vi "总磷氨氮通讯.vi"() -> ()   [LabVIEW 2016, in "斯坦道仪器.lvlib"]
uses:
  <vilib>/Plasmionique/MB Master/MB_Master_Serial/MB_Master_Serial.lvclass
  D:/Program Files (x86)/National Instruments/LabVIEW 2016/vi.lib/Plasmionique/MB Master/MB_Master/MB_Master.lvclass
  <vilib>/Utility/config.llb/Write Key (Boolean).vi
  <vilib>/Utility/config.llb/Write Key (String).vi
  <vilib>/Utility/config.llb/Read Key (Boolean).vi
  <vilib>/Utility/config.llb/Read Key (String).vi
  <vilib>/Plasmionique/MB Master/MB_Master/MB_Master.lvclass
  <vilib>/Utility/config.llb/NI_LVConfig.lvlib
  <vilib>/Plasmionique/MB Master/MB Master.lvlib
  <vilib>/ptbypt/NI_PtbyPt.lvlib
panel:
  out "量程":u16
  out "序列号":string
  out "状态告警区":T1
  out "测量数据区":T2 {"单位" items=["ug/L", "mg/L", "ppm", "mg/m3", "cm", "ppb", "ug/m3", "%", "nmol/mol", "umol/mol", "MPN/L", "MPN/100ml", "ng/m3", "NTU", "无量纲", "ms/cm", "us/cm", "℃", "mV", "万个/L"]}
  out "status":bool
  out "关键参数区":T3
  in  "读关键参数区":bool
  in  "读状态告警区":bool
  in  "读测量数据区":bool
  in  "站号":u16(ring) items=["总磷"=1, "氨氮"=3]
  in  "停止":bool
  in  "启动":bool
  in  "控制命令":u16(ring) items=["启动测量"=1, "标样核查"=2, "零点核查"=3, "跨度核查"=4, "空白测试"=5, "平行样测试"=6, "加标回收"=7, "空白校准"=8, "标样校准"=9, "初始化（清洗）"=10, "停止测试"=11, "仪器重启"=12, "校时"=13, "模式设置"=14, "测量间隔设置"=15]
  in  "控制命令参数":u16[](array[numeric]) format="%04xH"
  in  "VISA Resource":refnum<visa-resource-name>
  in  "启用模块":bool
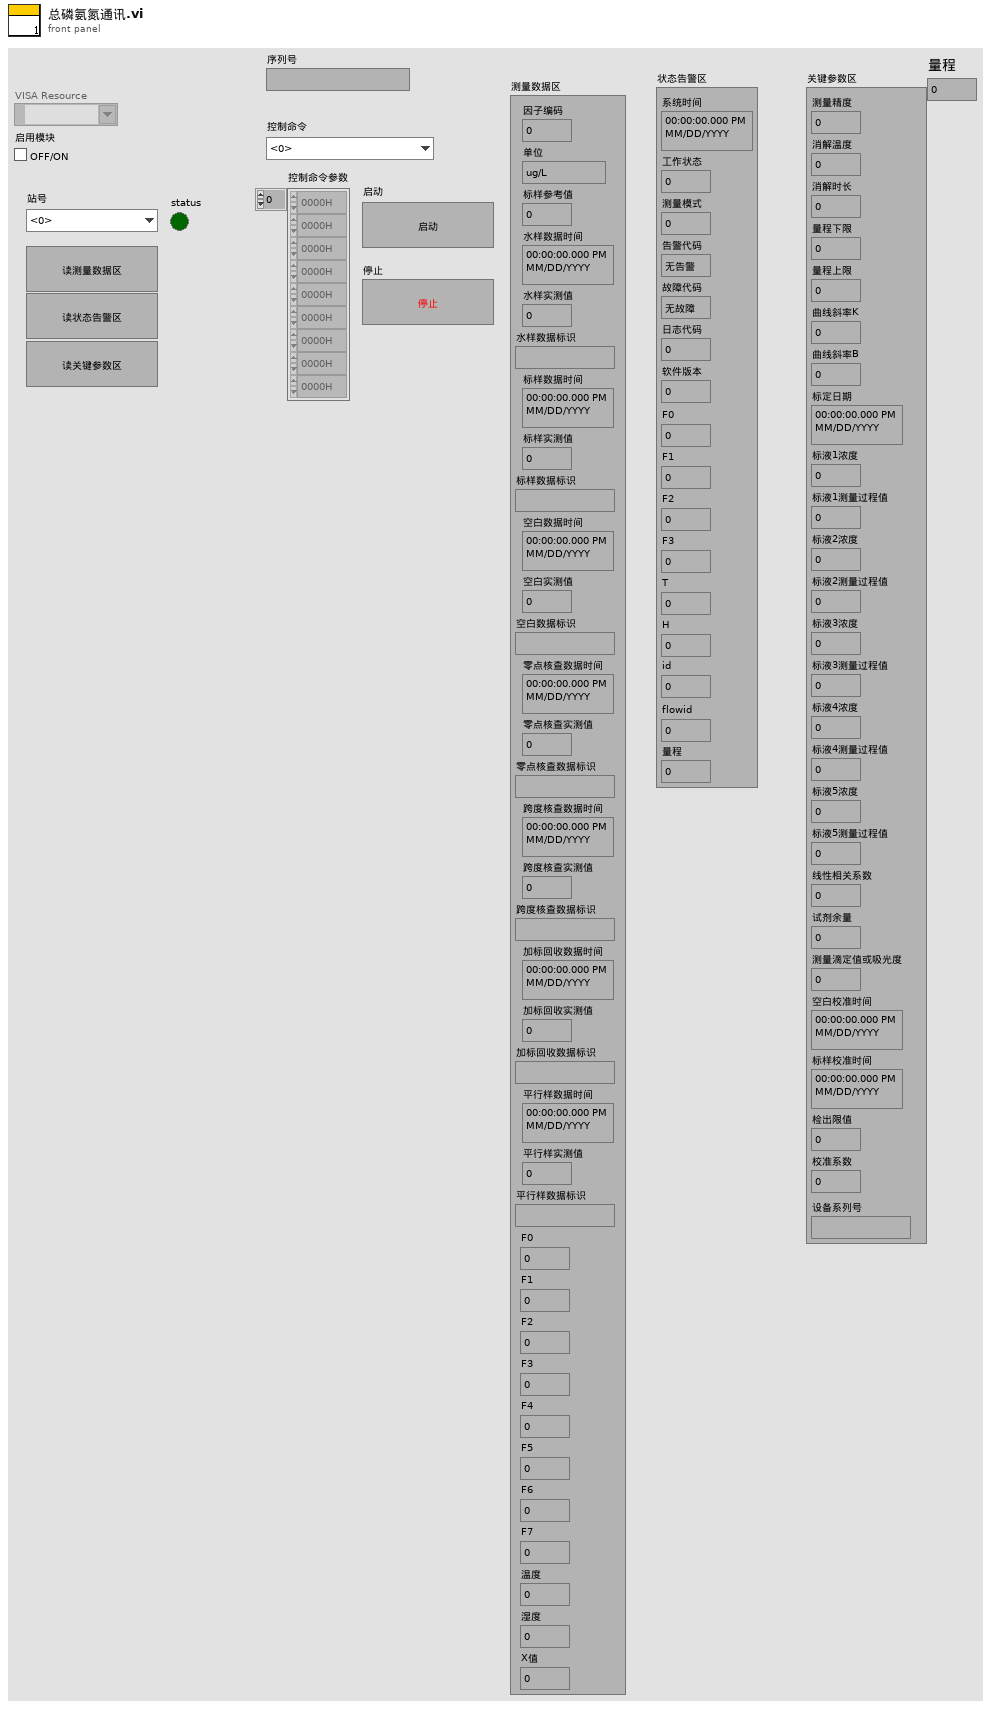
[diagram p1: front panel]
types:
  T1 = cluster{"系统时间":timestamp, "工作状态":u16, "测量模式":u16, "告警代码":enum16{"无告警", "缺试剂告警", "缺水样告警", "缺蒸馏水告警", "缺标液告警", "仪表漏液告警", "标定异常告警", "超量程告警", "加热异常", "低试剂预警", "超上限告警", "超下限告警", "仪表内部其他异常", "滴定异常告警", "电极异常告警", "量程切换告警", "参数设置告警", "PH电极电位异常", "电导率电极异常", "浊度光度异常", "溶解氧电极异常", "溶解氧光强异常", "温度异常告警", "PH异常告警", "溶解氧异常告警", "电导率异常告警", "浊度异常告警", "叶绿素异常告警", "藻密度异常告警", "蓝绿藻异常告警", "ORP异常告警", "氨氮异常告警", "清洁刷异常告警", "SD卡异常告警", "蓝牙异常告警", "Wifi异常告警", "流程异常告警"}, "故障代码":enum16{"无故障", "电机故障", "温度故障", "通讯故障", "滴定故障"}, "日志代码":u16, "软件版本":u16, "F0":sgl, "F1":sgl, "F2":sgl, "F3":sgl, "T":sgl, "H":sgl, "id":u16, "flowid":u16, "量程":u16}
  T2 = cluster{"因子编码":u32, "单位":u16, "标样参考值":sgl, "水样数据时间":timestamp, "水样实测值":sgl, "水样数据标识":string, "标样数据时间":timestamp, "标样实测值":sgl, "标样数据标识":string, "空白数据时间":timestamp, "空白实测值":sgl, "空白数据标识":string, "零点核查数据时间":timestamp, "零点核查实测值":sgl, "零点核查数据标识":string, "跨度核查数据时间":timestamp, "跨度核查实测值":sgl, "跨度核查数据标识":string, "加标回收数据时间":timestamp, "加标回收实测值":sgl, "加标回收数据标识":string, "平行样数据时间":timestamp, "平行样实测值":sgl, "平行样数据标识":string, "F0":sgl, "F1":sgl, "F2":sgl, "F3":sgl, "F4":sgl, "F5":sgl, "F6":sgl, "F7":sgl, "温度":sgl, "湿度":sgl, "X值":sgl}
  T3 = cluster{"测量精度":u16, "消解温度":u16, "消解时长":u16, "量程下限":sgl, "量程上限":sgl, "曲线斜率K":sgl, "曲线斜率B":sgl, "标定日期":timestamp, "标液1浓度":sgl, "标液1测量过程值":sgl, "标液2浓度":sgl, "标液2测量过程值":sgl, "标液3浓度":sgl, "标液3测量过程值":sgl, "标液4浓度":sgl, "标液4测量过程值":sgl, "标液5浓度":sgl, "标液5测量过程值":sgl, "线性相关系数":sgl, "试剂余量":u32, "测量滴定值或吸光度":sgl, "空白校准时间":timestamp, "标样校准时间":timestamp, "检出限值":sgl, "校准系数":sgl, "设备系列号":string}
  T4 = cluster{"系统时间":timestamp, "工作状态":enum16{"空闲", "水样测试", "标样核查", "零点核查", "跨度核查", "空白测试", "平行样测试", "加标回收", "空白校准", "标样校准", "初始化（清洗）"}, "测量模式":enum16{"待机", "连续模式", "周期模式", "定点模式", "受控模式", "手动模式"}, "告警代码":enum16{"无告警", "缺试剂告警", "缺水样告警", "缺蒸馏水告警", "缺标液告警", "仪表漏液告警", "标定异常告警", "超量程告警", "加热异常", "低试剂预警", "超上限告警", "超下限告警", "仪表内部其他异常", "滴定异常告警", "电极异常告警", "量程切换告警", "参数设置告警", "PH电极电位异常", "电导率电极异常", "浊度光度异常", "溶解氧电极异常", "溶解氧光强异常", "温度异常告警", "PH异常告警", "溶解氧异常告警", "电导率异常告警", "浊度异常告警", "叶绿素异常告警", "藻密度异常告警", "蓝绿藻异常告警", "ORP异常告警", "氨氮异常告警", "清洁刷异常告警", "SD卡异常告警", "蓝牙异常告警", "Wifi异常告警", "流程异常告警"}, "故障代码":enum16{"无故障", "电机故障", "温度故障", "通讯故障", "滴定故障"}, "日志代码":u16, "软件版本":u16, "F0":sgl, "F1":sgl, "F2":sgl, "F3":sgl, "T":sgl, "H":sgl, "id":u16, "flowid":u16, "量程":u16}
  T5 = typedef "NI_LVConfig.lvlib/Config Data RefNum.ctl" = refnum<k1>
  T6 = enum8{"Enabled", "Disabled", "Disabled and Grayed Out"}
  T7 = cluster{"baud rate (bps)":u32, "stop bits":u16, "parity":u16, "flow control":u16, "timeout":u32, "retries":i32}
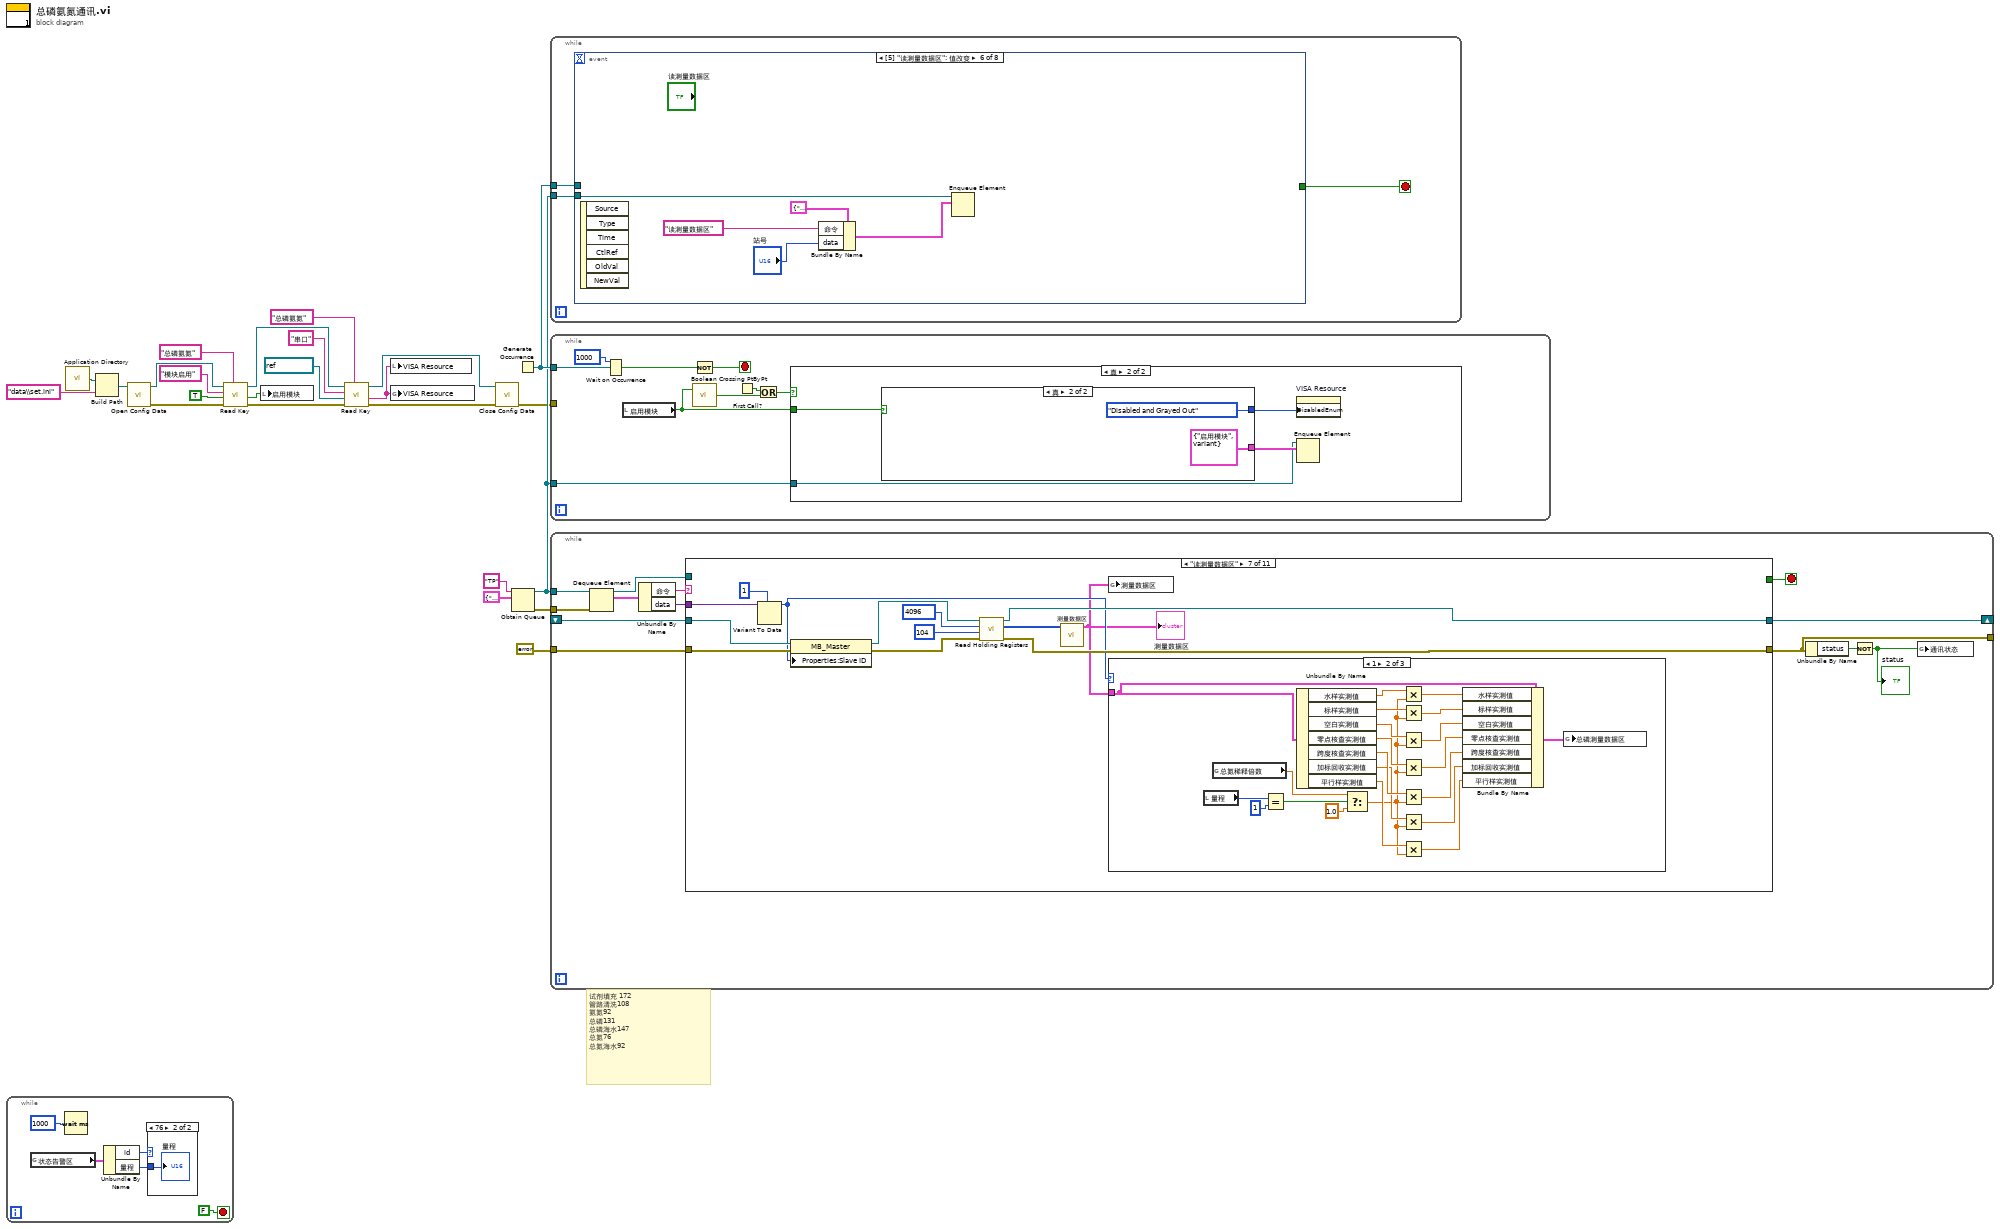
[diagram p0: block diagram]
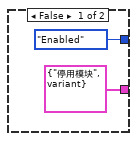
[diagram p4: hidden frame]
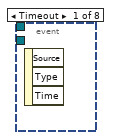
[diagram p5: hidden frame]
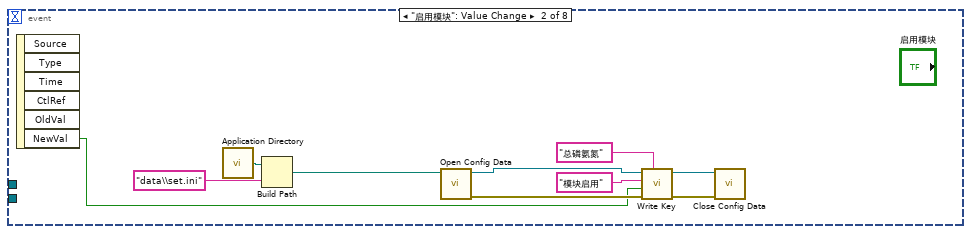
[diagram p6: hidden frame]
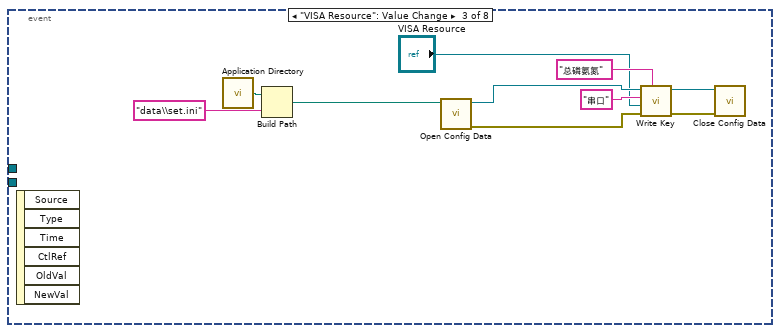
[diagram p7: hidden frame]
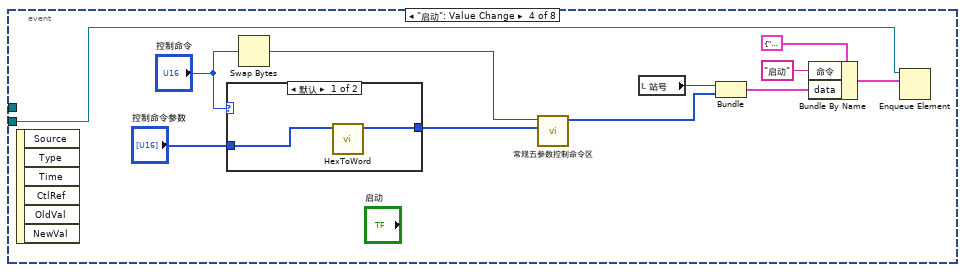
[diagram p8: hidden frame]
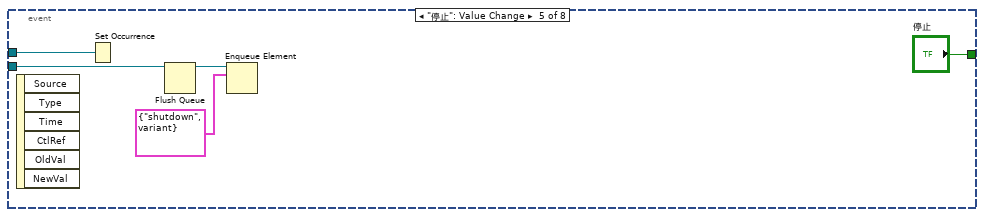
[diagram p10: hidden frame]
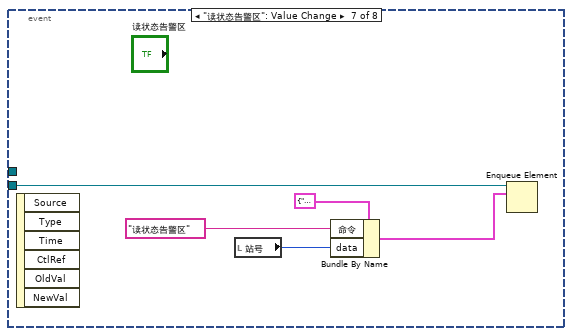
[diagram p11: hidden frame]
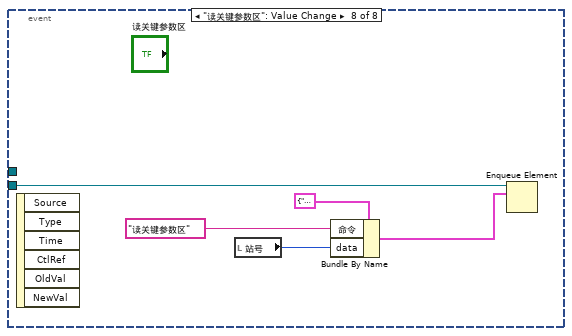
[diagram p12: hidden frame]
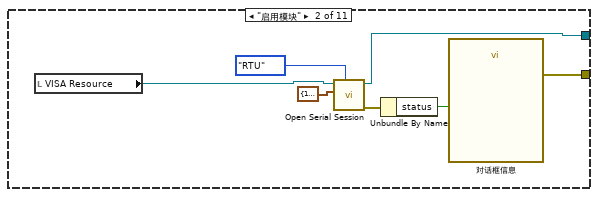
[diagram p14: hidden frame]
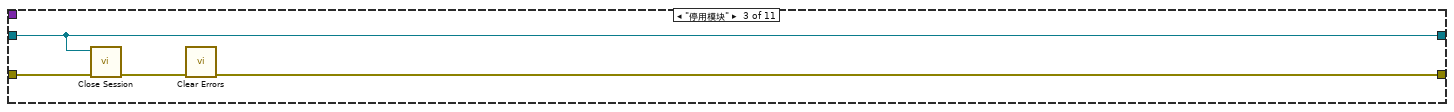
[diagram p15: hidden frame]
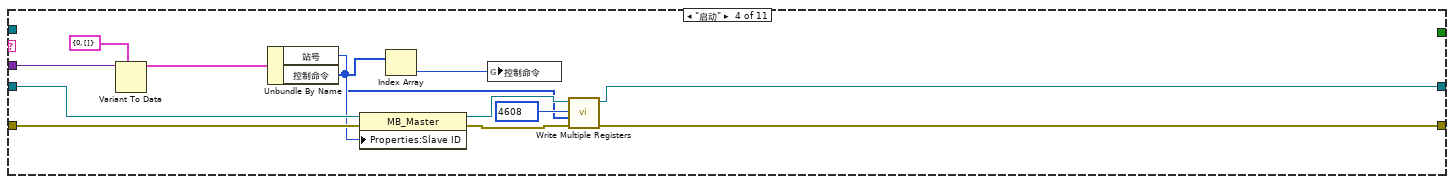
[diagram p16: hidden frame]
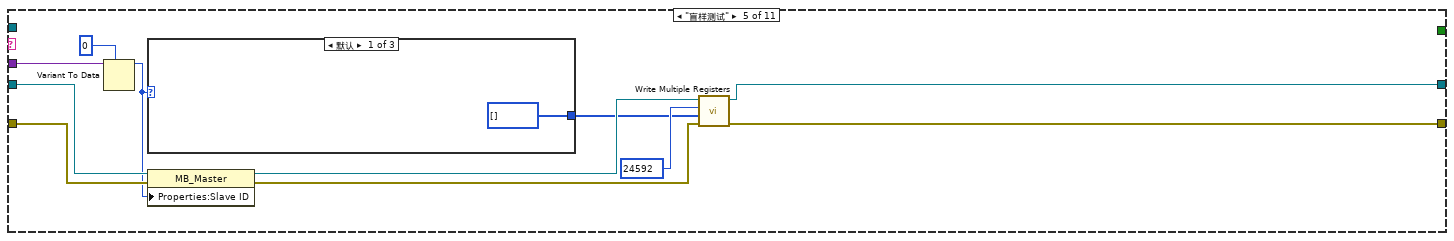
[diagram p17: hidden frame]
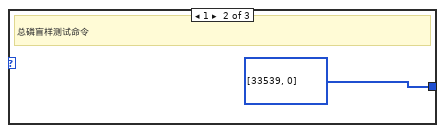
[diagram p18: hidden frame]
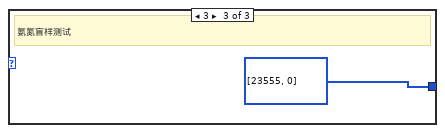
[diagram p19: hidden frame]
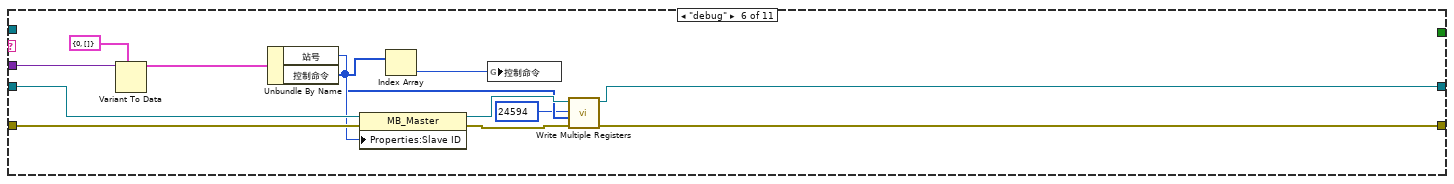
[diagram p20: hidden frame]
diagram:
  # "试剂填充 172 \n管路清洗108\n氨氮92\n总磷131\n总磷海水147\n总氮76\n总氮海水92"
  n1 = while {
    stop <- FALSE stop-if-true
    n2 = global read "VAR总磷氨氮全局变量.vi" "状态告警区"() -> (w29:T4)
    n3 = Wait (ms)(milliseconds to wait=u32 1000 ("等待时间（毫秒）")) -> ()  [unwired: 1 out]
    n4 = Unbundle By Name(w29) -> ("id"=w26:u16, "量程"=w25:u16)
    n5 = case shown="76" w26 {
      tunnel: w25 -> [_ w30]
      frame 0, Default {
      }
      frame 76 {
        "量程" <- w30
      }
    }
  }
  n6 = call <vilib>:"Application Directory.vi"() -> ("Application Directory"=w12:path)
  n7 = Build Path(base path=w12, name or relative path="data\\set.ini" ("名称或相对路径")) -> (appended path=w13:path)
  n8 = call <vilib>:"Open Config Data.vi"("configuration file path"=w13) -> ("error out"=w18:errorcluster, "refnum"=w17:T5)  [unwired: 8 in, 1 out]
  n9 = call-poly <vilib>:"Read Key.vi"("section"="总磷氨氮", "error in (no error)"=w18, "default value"=TRUE ("启用模块"), "key"="模块启用", "refnum"=w17) -> ("error out"=w6:errorcluster, "value"=w9:bool, "refnum out"=w8:T5)  [unwired: 3 in, 1 out]
  n10 = local write "启用模块"(w9) -> ()
  n11 = call-poly <vilib>:"Read Key.vi"("section"="总磷氨氮", "error in (no error)"=w6, "default value"=refnum<visa-resource-name> "COM4" ("VISA Resource"), "key"="串口", "refnum"=w8) -> ("error out"=w5:errorcluster, "value"=w1:string, "refnum out"=w7:T5)  [unwired: 3 in, 1 out]
  n12 = local write "VISA Resource"(w1) -> ()
  n13 = global write "VAR总磷氨氮全局变量.vi" "VISA Resource"(w1) -> ()
  n14 = call <vilib>:"Close Config Data.vi"("error in (no error)"=w5, "refnum"=w7) -> ("error out"=w10:errorcluster)  [unwired: 8 in, 1 out]
  n15 = Obtain Queue(name (unnamed)="TP" ("名称（未命名）"), element data type=cluster{"命令":string, "data":variant} {"命令"="", "data"=variant}) -> (queue out=w19:refnum<queue>, error out=w22:errorcluster)  [unwired: 3 in, 1 out]
  n16 = Generate Occurrence() -> (w20:refnum<k4>)
  n17 = while {
    tunnel: w19 -> [w33]
    tunnel: w20 -> [w31]
    stop <- w32 stop-if-true
    n18 = event shown="[5] \"读测量数据区\": 值改变" {
      selector: _ -> [_ _ _ _ _ _ _ _]
      dyn-events: _ -> [_ _ _ _ _ _ _ _]
      timeout: _ -> [_ _ _ _ _ _ _ _]
      tunnel: w33 -> [_ _ _ w64 w71 w77 w82 w87]
      tunnel: [_ _ _ _ "停止" _ _ _] -> w32
      tunnel: w31 -> [_ _ _ _ w68 _ _ _]
      event Timeout {
        n19 = event-data() -> ()  [unwired: 1 in, 3 out]
      }
      event "启用模块": Value Change {
        n20 = event-data() -> ("NewVal"=w34:bool)  [unwired: 1 in, 5 out]
        n21 = call <vilib>:"Application Directory.vi"() -> ("Application Directory"=w36:path)
        n22 = Build Path(base path=w36, name or relative path="data\\set.ini" ("名称或相对路径")) -> (appended path=w37:path)
        n23 = call <vilib>:"Open Config Data.vi"("configuration file path"=w37) -> ("error out"=w43:errorcluster, "refnum"=w42:T5)  [unwired: 8 in, 1 out]
        n24 = call-poly <vilib>:"Write Key.vi"("section"="总磷氨氮", "error in (no error)"=w43, "value"=w34, "key"="模块启用", "refnum"=w42) -> ("error out"=w39:errorcluster, "refnum out"=w35:T5)  [unwired: 4 in, 1 out]
        n25 = call <vilib>:"Close Config Data.vi"("error in (no error)"=w39, "refnum"=w35) -> ()  [unwired: 8 in, 2 out]
      }
      event "VISA Resource": Value Change {
        n26 = event-data() -> ()  [unwired: 1 in, 6 out]
        n27 = call <vilib>:"Application Directory.vi"() -> ("Application Directory"=w46:path)
        n28 = Build Path(base path=w46, name or relative path="data\\set.ini" ("名称或相对路径")) -> (appended path=w47:path)
        n29 = call <vilib>:"Open Config Data.vi"("configuration file path"=w47) -> ("error out"=w53:errorcluster, "refnum"=w52:T5)  [unwired: 8 in, 1 out]
        n30 = call-poly <vilib>:"Write Key.vi"("section"="总磷氨氮", "error in (no error)"=w53, "value"="VISA Resource", "key"="串口", "refnum"=w52) -> ("error out"=w49:errorcluster, "refnum out"=w45:T5)  [unwired: 4 in, 1 out]
        n31 = call <vilib>:"Close Config Data.vi"("error in (no error)"=w49, "refnum"=w45) -> ()  [unwired: 8 in, 2 out]
      }
      event "启动": Value Change {
        n32 = event-data() -> ()  [unwired: 1 in, 6 out]
        n33 = case shown="默认" "控制命令" {
          tunnel: "控制命令参数" -> [w66 w67]
          tunnel: [w65 w67] -> w54
          frame Default {
            n34 = call "HexToWord.vi"("数组"=w66) -> ("WORD"=w65:u16[])  [unwired: 10 in]
          }
          frame 13 {
          }
        }
        n35 = Swap Bytes(anything="控制命令") -> (byte swapped=w57:u16)
        n36 = call "常规五参数控制命令区.vi"("控制命令参数"=w54, "控制命令"=w57) -> ("控制命令输出"=w60:u16[])  [unwired: 9 in]
        n37 = local read "站号"() -> (w59:u16)
        n38 = Bundle("站号"=w59, "控制命令输出"=w60) -> (w58:cluster{"站号":u16, "控制命令输出":u16[]})  [unwired: 1 in]
        n39 = Bundle By Name(cluster=cluster{"命令":string, "data":variant} {"命令"="", "data"=variant} ("元素"), "命令"="启动", "data"=w58) -> (w62:cluster{"命令":string, "data":variant})
        n40 = Enqueue Element(queue=w64, element=w62) -> ()  [unwired: 2 in, 3 out]
      }
      event "停止": Value Change {
        n41 = event-data() -> ()  [unwired: 1 in, 6 out]
        n42 = Set Occurrence(w68) -> ()
        n43 = Flush Queue(queue=w71) -> (queue out=w70:refnum<queue>)  [unwired: 1 in, 2 out]
        n44 = Enqueue Element(queue=w70, element=cluster{"命令":string, "data":variant} {"命令"="shutdown", "data"=variant} ("元素")) -> ()  [unwired: 2 in, 3 out]
      }
      event "读测量数据区": Value Change {
        n45 = event-data() -> ()  [unwired: 1 in, 6 out]
        n46 = Bundle By Name(cluster=cluster{"命令":string, "data":variant} {"命令"="", "data"=variant} ("元素"), "命令"="读测量数据区", "data"="站号") -> (w75:cluster{"命令":string, "data":variant})
        n47 = Enqueue Element(queue=w77, element=w75) -> ()  [unwired: 2 in, 3 out]
      }
      event "读状态告警区": Value Change {
        n48 = event-data() -> ()  [unwired: 1 in, 6 out]
        n49 = local read "站号"() -> (w78:u16)
        n50 = Bundle By Name(cluster=cluster{"命令":string, "data":variant} {"命令"="", "data"=variant} ("元素"), "命令"="读状态告警区", "data"=w78) -> (w80:cluster{"命令":string, "data":variant})
        n51 = Enqueue Element(queue=w82, element=w80) -> ()  [unwired: 2 in, 3 out]
      }
      event "读关键参数区": Value Change {
        n52 = event-data() -> ()  [unwired: 1 in, 6 out]
        n53 = local read "站号"() -> (w83:u16)
        n54 = Bundle By Name(cluster=cluster{"命令":string, "data":variant} {"命令"="", "data"=variant} ("元素"), "命令"="读关键参数区", "data"=w83) -> (w85:cluster{"命令":string, "data":variant})
        n55 = Enqueue Element(queue=w87, element=w85) -> ()  [unwired: 2 in, 3 out]
      }
    }
  }
  n56 = while {
    tunnel: w20 -> [w96]
    tunnel: w19 -> [w91]
    tunnel: w10 -> [_]
    stop <- w93 stop-if-true
    n57 = Wait on Occurrence(2:w96, 3:1000 ("毫秒超时(-1)")) -> (0:w94:bool)  [unwired: 1 in]
    n58 = local read "启用模块"() -> (w92:bool)
    n59 = Not(x=w94) -> (.not. x?=w93:bool)
    n60 = call <vilib>:"Boolean Crossing PtByPt.vi"("input"=w92) -> ("crossing"=w89:bool)  [unwired: 2 in]
    n61 = First Call?() -> (First Call?: T/F=w90:bool)
    n62 = Or(x=w90, y=w89) -> (x .or. y?=w88:bool)
    n63 = case shown="真" w88 {
      tunnel: w92 -> [_ w99]
      tunnel: w91 -> [_ w98]
      frame False {
      }
      frame True {
        n64 = case shown="真" w99 {
          tunnel: [cluster{"命令":string, "data":variant} {"命令"="停用模块", "data"=variant} ("元素") cluster{"命令":string, "data":variant} {"命令"="启用模块", "data"=variant} ("元素")] -> w100
          tunnel: [T6."Enabled" ("禁用") T6."Disabled and Grayed Out" ("禁用")] -> w97
          frame False {
          }
          frame True {
          }
        }
        n65 = property on="VISA Resource" class="VISAName"("DisabledEnum"=w97) -> ()  [unwired: 2 in, 2 out]
        n66 = Enqueue Element(queue=w98, element=w100) -> ()  [unwired: 2 in, 3 out]
      }
    }
  }
  n67 = while {
    tunnel: w19 -> [w117]
    tunnel: w22 -> [w116]
    shift-right: [w114] -> _
    shift-left: _ -> [w113]
    tunnel: errorcluster {"status"=FALSE, "code"=0, "source"=""} ("error out") -> [w112]
    tunnel: [w107] -> _
    stop <- w115 stop-if-true
    n68 = Dequeue Element(queue=w117, error in (no error)=w116) -> (queue out=w108:refnum<queue>, element=w110:cluster{"命令":string, "data":variant})  [unwired: 1 in, 2 out]
    n69 = Unbundle By Name(w110) -> ("命令"=w111:string, "data"=w109:variant)
    n70 = case shown="\"读测量数据区\"" w111 {
      tunnel: w109 -> [_ _ _ w140 w151 w168 w178 w209 w224 w238 _]
      tunnel: w108 -> [_ _ _ _ _ _ _ _ _ _ w251]
      tunnel: [_ _ _ _ _ _ _ _ _ _ TRUE] -> w115
      tunnel: [w118 w126 w127 w143 w154 w170 w182 w218 w231 w245 w247] -> w114
      tunnel: [w119 w121 w128 w142 w153 w169 w183 w219 w232 w246 w248] -> w107
      tunnel: w113 -> [w118 _ w127 w139 w150 w167 w177 w212 w227 w241 w247]
      tunnel: w112 -> [w119 _ w130 w136 w147 w164 w175 w213 w228 w242 w249]
      frame Default {
      }
      frame "启用模块" {
        n71 = local read "VISA Resource"() -> (w120:refnum<visa-resource-name>)
        n72 = call <vilib>:"Open Serial Session.vi"("Mode (RTU)"=enum16{"RTU", "ASCII"}."RTU", "Serial Config"=T7 {"baud rate (bps)"=115200, "stop bits"=10, "parity"=0, "flow control"=0, "timeout"=1000, "retries"=1}, "VISA Resource"=w120) -> ("Error out"=w122:errorcluster, "MB_Serial session"=w126:refnum<class "MB_Master_Serial.lvclass">)  [unwired: 7 in]
        n73 = Unbundle By Name(w122) -> ("status"=w123:bool)
        n74 = call "对话框信息"("Enable"=w123) -> ("error out"=w121:errorcluster)  [unwired: 9 in, 1 out]
      }
      frame "停用模块" {
        n75 = call-dynamic "Close Session.vi"("error in (no error)"=w130, "MB session in"=w127) -> ("error out"=w129:errorcluster)  [unwired: 9 in]
        n76 = call <vilib>:"Clear Errors.vi"("error in (no error)"=w129) -> ("error out"=w128:errorcluster)  [unwired: 5 in, 1 out]
      }
      frame "启动" {
        n77 = Variant To Data(type=cluster{"站号":u16, "控制命令":u16[]} {"站号"=0, "控制命令"=[]} ("输出簇"), Variant=w140) -> (data=w134:cluster{"站号":u16, "控制命令":u16[]})  [unwired: 1 in, 1 out]
        n78 = Unbundle By Name(w134) -> ("站号"=w133:u16, "控制命令"=w131:u16[])
        n79 = property class="MB_Master"(reference=w139, error in=w136, "Properties:Slave ID"=w133) -> (reference out=w138:refnum<class "MB_Master.lvclass">, error out=w137:errorcluster)
        n80 = Index Array(array=w131) -> (element=w132:u16)  [unwired: 1 in]
        n81 = global write "VAR总磷氨氮全局变量.vi" "控制命令"(w132) -> ()
        n82 = call <vilib>:"Write Multiple Registers.vi"("error in (no error)"=w137, "values"=w131, "starting address"=u16 4608, "MB session in"=w138) -> ("error out"=w142:errorcluster, "MB session out"=w143:refnum<class "MB_Master.lvclass">)  [unwired: 6 in]
      }
      frame "盲样测试" {
        n83 = Variant To Data(type=0, Variant=w151) -> (data=w144:i32)  [unwired: 1 in, 1 out]
        n84 = case shown="默认" w144 {
          tunnel: [u16[] [] ("values") u16[] [33539, 0] ("values") u16[] [23555, 0] ("values")] -> w146
          frame Default {
          }
          frame 1 {
            # "总磷盲样测试命令"
          }
          frame 3 {
            # "氨氮盲样测试"
          }
        }
        n85 = property class="MB_Master"(reference=w150, error in=w147, "Properties:Slave ID"=w144) -> (reference out=w149:refnum<class "MB_Master.lvclass">, error out=w148:errorcluster)
        n86 = call <vilib>:"Write Multiple Registers.vi"("error in (no error)"=w148, "values"=w146, "starting address"=u16 24592, "MB session in"=w149) -> ("error out"=w153:errorcluster, "MB session out"=w154:refnum<class "MB_Master.lvclass">)  [unwired: 6 in]
      }
      frame "debug" {
        n87 = Variant To Data(type=cluster{"站号":u16, "控制命令":u16[]} {"站号"=0, "控制命令"=[]} ("输出簇"), Variant=w168) -> (data=w162:cluster{"站号":u16, "控制命令":u16[]})  [unwired: 1 in, 1 out]
        n88 = Unbundle By Name(w162) -> ("站号"=w161:u16, "控制命令"=w159:u16[])
        n89 = property class="MB_Master"(reference=w167, error in=w164, "Properties:Slave ID"=w161) -> (reference out=w166:refnum<class "MB_Master.lvclass">, error out=w165:errorcluster)
        n90 = Index Array(array=w159) -> (element=w160:u16)  [unwired: 1 in]
        n91 = global write "VAR总磷氨氮全局变量.vi" "控制命令"(w160) -> ()
        n92 = call <vilib>:"Write Multiple Registers.vi"("error in (no error)"=w165, "values"=w159, "starting address"=u16 24594, "MB session in"=w166) -> ("error out"=w169:errorcluster, "MB session out"=w170:refnum<class "MB_Master.lvclass">)  [unwired: 6 in]
      }
      frame "读测量数据区" {
        n93 = Variant To Data(type=u8 1 ("Slave ID"), Variant=w178) -> (data=w172:u8)  [unwired: 1 in, 1 out]
        n94 = property class="MB_Master"(reference=w177, error in=w175, "Properties:Slave ID"=w172) -> (reference out=w176:refnum<class "MB_Master.lvclass">, error out=w174:errorcluster)
        n95 = call <vilib>:"Read Holding Registers.vi"("error in (no error)"=w174, "quantity"=u16 104, "starting address"=u16 4096, "MB session in"=w176) -> ("error out"=w183:errorcluster, "Registers"=w173:u16[], "MB session out"=w182:refnum<class "MB_Master.lvclass">)  [unwired: 5 in]
        n96 = call "测量数据区.vi"("数组"=w173) -> ("测量数据区"=w171:T2)  [unwired: 10 in]
        "测量数据区" <- w171
        n97 = global write "VAR总磷氨氮全局变量.vi" "测量数据区"(w171) -> ()
        n98 = case shown="1" w172 {
          tunnel: w171 -> [_ w205 w206]
          frame 0, Default {
          }
          frame 1 {
            n99 = local read "量程"() -> (w186:u16)
            n100 = global read "VAR总磷氨氮全局变量.vi" "总氮稀释倍数"() -> (w189:dbl)
            n101 = Equal?(x=w186, y=u16 1) -> (x = y?=w184:bool)
            n102 = Unbundle By Name(w205) -> ("水样实测值"=w203:sgl, "标样实测值"=w201:sgl, "空白实测值"=w199:sgl, "零点核查实测值"=w197:sgl, "跨度核查实测值"=w195:sgl, "加标回收实测值"=w193:sgl, "平行样实测值"=w191:sgl)
            n103 = Select(t=w189, s=w184, f=1.0) -> (s? t:f=w187:dbl)
            n104 = Multiply(x=w203, y=w187) -> (x*y=w202:dbl)
            n105 = Multiply(x=w201, y=w187) -> (x*y=w200:dbl)
            n106 = Multiply(x=w199, y=w187) -> (x*y=w198:dbl)
            n107 = Multiply(x=w197, y=w187) -> (x*y=w196:dbl)
            n108 = Multiply(x=w195, y=w187) -> (x*y=w194:dbl)
            n109 = Multiply(x=w193, y=w187) -> (x*y=w192:dbl)
            n110 = Multiply(x=w191, y=w187) -> (x*y=w190:dbl)
            n111 = Bundle By Name(cluster=w205, "水样实测值"=w202, "标样实测值"=w200, "空白实测值"=w198, "零点核查实测值"=w196, "跨度核查实测值"=w194, "加标回收实测值"=w192, "平行样实测值"=w190) -> (w204:T2)
            n112 = global write "VAR总磷氨氮全局变量.vi" "总磷测量数据区"(w204) -> ()
          }
          frame 2 {
            n113 = global write "VAR总磷氨氮全局变量.vi" "总氮测量数据区"(w206) -> ()
          }
        }
      }
      frame "读状态告警区" {
        n114 = Variant To Data(type=u8 1 ("Slave ID"), Variant=w209) -> (data=w214:u8)  [unwired: 1 in, 1 out]
        n115 = property class="MB_Master"(reference=w212, error in=w213, "Properties:Slave ID"=w214) -> (reference out=w211:refnum<class "MB_Master.lvclass">, error out=w210:errorcluster)
        n116 = call <vilib>:"Read Holding Registers.vi"("error in (no error)"=w210, "quantity"=u16 24, "starting address"=u16 4224, "MB session in"=w211) -> ("error out"=w219:errorcluster, "Registers"=w208:u16[], "MB session out"=w218:refnum<class "MB_Master.lvclass">)  [unwired: 5 in]
        n117 = call "状态告警区.vi"("数组"=w208) -> ("状态告警区"=w207:T4)  [unwired: 10 in]
        "状态告警区" <- w207
        n118 = global write "VAR总磷氨氮全局变量.vi" "状态告警区"(w207) -> ()
      }
      frame "读关键参数区" {
        n119 = Variant To Data(type=u8 1 ("Slave ID"), Variant=w224) -> (data=w222:u8)  [unwired: 1 in, 1 out]
        n120 = property class="MB_Master"(reference=w227, error in=w228, "Properties:Slave ID"=w222) -> (reference out=w226:refnum<class "MB_Master.lvclass">, error out=w225:errorcluster)
        n121 = call <vilib>:"Read Holding Registers.vi"("error in (no error)"=w225, "quantity"=u16 19, "starting address"=u16 4256, "MB session in"=w226) -> ("error out"=w232:errorcluster, "Registers"=w221:u16[], "MB session out"=w231:refnum<class "MB_Master.lvclass">)  [unwired: 5 in]
        n122 = call "关键参数区.vi"("数组"=w221) -> ("关键参数区"=w220:T3)  [unwired: 10 in]
        "关键参数区" <- w220
        n123 = global write "VAR总磷氨氮全局变量.vi" "关键参数区"(w220) -> ()
      }
      frame "读序列号" {
        n124 = Variant To Data(type=u8 1 ("Slave ID"), Variant=w238) -> (data=w236:u8)  [unwired: 1 in, 1 out]
        n125 = property class="MB_Master"(reference=w241, error in=w242, "Properties:Slave ID"=w236) -> (reference out=w240:refnum<class "MB_Master.lvclass">, error out=w239:errorcluster)
        n126 = call <vilib>:"Read Holding Registers.vi"("error in (no error)"=w239, "quantity"=u16 6, "starting address"=u16 3, "MB session in"=w240) -> ("error out"=w246:errorcluster, "Registers"=w235:u16[], "MB session out"=w245:refnum<class "MB_Master.lvclass">)  [unwired: 5 in]
        n127 = call "HexToString.vi"("数组"=w235) -> ("STRING"=w234:string[])  [unwired: 10 in]
        n128 = Index Array(array=w234) -> (element=w233:string)  [unwired: 1 in]
        "序列号" <- w233
        n129 = global write "VAR总磷氨氮全局变量.vi" "序列号"(w233) -> ()
      }
      frame "shutdown" {
        n130 = call-dynamic "Close Session.vi"("error in (no error)"=w249, "MB session in"=w247) -> ("error out"=w248:errorcluster)  [unwired: 9 in]
        n131 = Flush Queue(queue=w251) -> (queue out=w250:refnum<queue>)  [unwired: 1 in, 2 out]
        n132 = Release Queue(queue=w250) -> ()  [unwired: 2 in, 3 out]
      }
    }
    n133 = Unbundle By Name(w107) -> ("status"=w106:bool)
    n134 = Not(x=w106) -> (.not. x?=w105:bool)
    "status" <- w105
    n135 = global write "VAR总磷氨氮全局变量.vi" "通讯状态"(w105) -> ()
  }
